vi "DualCam Field Angle.vi"() -> (0 "LTarget Dist":dbl, 1 "Field-Rel LTarget Angle":dbl, 3 "Gyro Angle":dbl, 4 "Found?":bool)   [LabVIEW 2013]
panel:
  in  "R Dist":dbl
  in  "Goal Apartness":dbl=18.9
  in  "R(B) Angle":dbl
  in  "R Found?":bool
  in  "L(A) Angle":dbl
  in  "L Found?":bool
  in  "L Dist":dbl
  out "A Angle":dbl
  out "C Angle":dbl
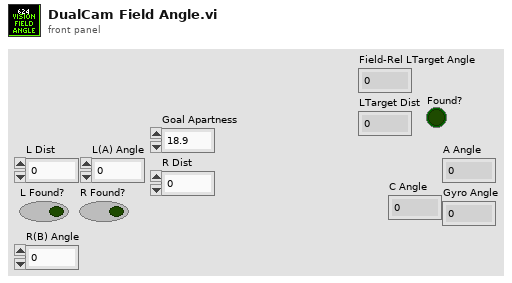
[diagram p1: front panel]
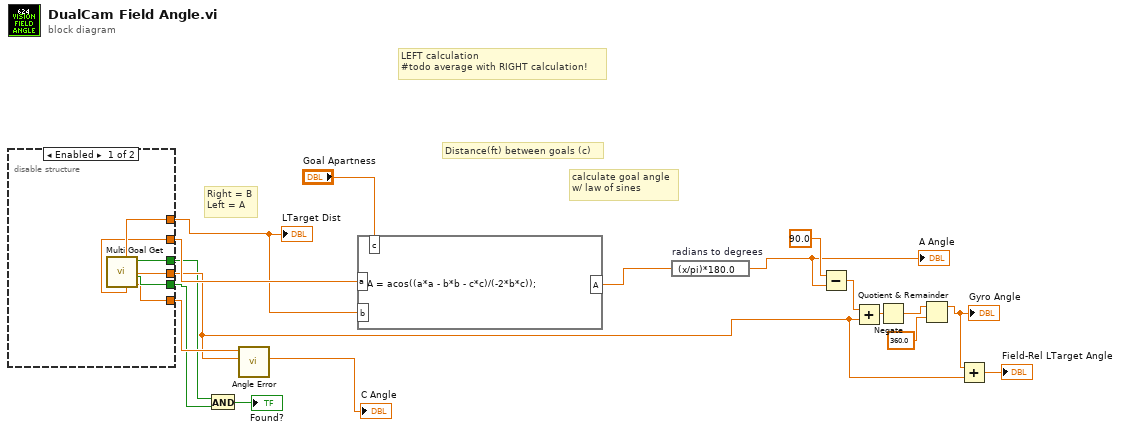
[diagram p0: block diagram]
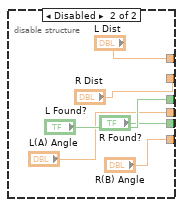
[diagram p2: hidden frame]
diagram:
  # "LEFT calculation\n#todo average with RIGHT calculation!"
  # "calculate goal angle\nw/ law of sines"
  # "Distance(ft) between goals (c)"
  # "Right = B\nLeft = A"
  n1 = disable-structure shown="Enabled" {
    disable-tunnel: [w24 "L Found?"] -> w3
    disable-tunnel: [w23 "R Found?"] -> w2
    disable-tunnel: [w22 "R(B) Angle"] -> w15
    disable-tunnel: [w21 "L Dist"] -> w4
    disable-tunnel: [w20 "L(A) Angle"] -> w6
    disable-tunnel: [w19 "R Dist"] -> w17
    frame Enabled {
      n2 = call "Multi Goal Get.vi"() -> ("R Robot-Rel X"=w22:dbl, "R Found?"=w23:bool, "L Robot-Rel X"=w20:dbl, "L Found?"=w24:bool, "R Dist"=w19:dbl, "L Dist"=w21:dbl)  [unwired: 4 in, 2 out]
    }
    frame Disabled {
    }
  }
  "LTarget Dist" <- w4
  n3 = And(x=w3, y=w2) -> (x .and. y?=→"Found?":bool)
  n4 = call "Angle Error.vi"("Angle"=w6, "Target Angle"=w15) -> ("Error"=→"C Angle":dbl)  [unwired: 9 in]
  n5 = formula code="A = acos((a*a - b*b - c*c)/(-2*b*c));"("a"=w17, "b"=w4, "c"="Goal Apartness") -> ("A"=w16:dbl)
  n6 = expression code="(x/pi)*180.0" "radians to degrees"(w16) -> (w12:dbl)
  "A Angle" <- w12
  n7 = Subtract(x=90.0, y=w12) -> (x-y=w11:dbl)
  n8 = Add(x=w11, y=w6) -> (x+y=w10:dbl)
  n9 = Negate(x=w10) -> (-x=w9:dbl)
  n10 = Quotient & Remainder(x=w9, y=360.0) -> (x-y*floor(x/y)=w7:dbl)  [unwired: 1 out]
  "Gyro Angle" <- w7
  n11 = Add(x=w7, y=w6) -> (x+y=→"Field-Rel LTarget Angle":dbl)
